vi "CountDown.vi"(10 "Cluster":T1) -> (2 "Cluster 2":T1)   [LabVIEW 2010]
uses:
  DataCluster.ctl
panel:
  out "Zero":bool
  out "Gauge":dbl(knob)
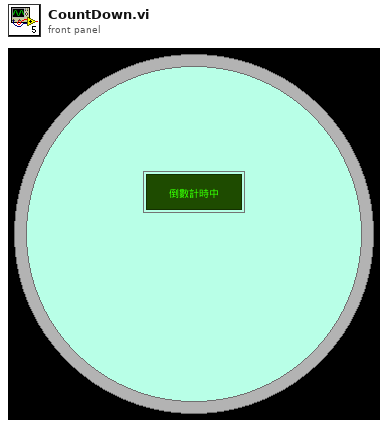
[diagram p1: front panel]
types:
  T1 = typedef "DataCluster.ctl" = cluster{"鬧鐘時間":timestamp, "鈴聲":path, "error ":errorcluster, "Min":dbl, "Sec":dbl, "鬧鐘作用":bool}
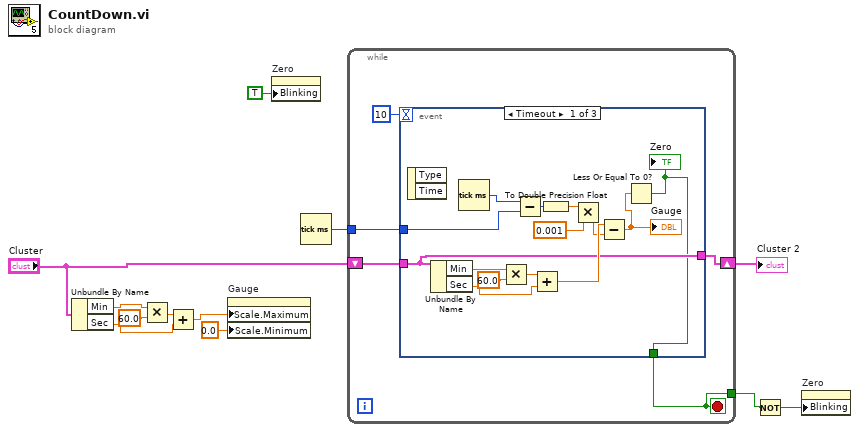
[diagram p0: block diagram]
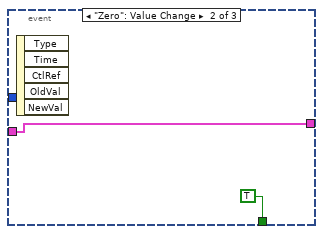
[diagram p2: hidden frame]
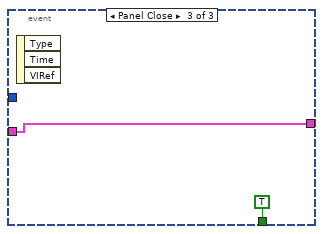
[diagram p3: hidden frame]
diagram:
  n1 = Unbundle By Name("Cluster") -> ("Min"=w4:dbl, "Sec"=w7:dbl)
  n2 = Multiply(x=w4, y=60.0) -> (x*y=w3:dbl)
  n3 = Add(x=w3, y=w7) -> (x+y=w2:dbl)
  n4 = property on="Gauge" class="Knob (strict)"("Scale.Maximum"=w2, "Scale.Minimum"=0.0 ("Scale.Range:Minimum")) -> ()  [unwired: 2 in, 2 out]
  n5 = property on="Zero" class="Bool (strict)"("Blinking"=TRUE) -> ()  [unwired: 2 in, 2 out]
  n6 = Tick Count (ms)() -> (millisecond timer value=w11:u32)
  n7 = while {
    shift-right: [w14] -> w10
    shift-left: "Cluster" -> [w16]
    tunnel: w11 -> [w15]
    tunnel: [w13] -> w8
    stop <- w13 stop-if-true
    n8 = event shown="[0] Timeout" {
      selector: _ -> [_ _ _]
      dyn-events: _ -> [_ _ _]
      timeout: 10 -> [_ _ _]
      tunnel: w16 -> [w20 w33 w35]
      tunnel: w15 -> [w26 _ _]
      tunnel: [w20 w33 w35] -> w14
      tunnel: [w18 TRUE TRUE] -> w13
      event Timeout {
        n9 = event-data() -> ()  [unwired: 1 in, 2 out]
        n10 = Unbundle By Name(w20) -> ("Min"=w31:dbl, "Sec"=w28:dbl)
        n11 = Tick Count (ms)() -> (millisecond timer value=w27:u32)
        n12 = Multiply(x=w31, y=60.0) -> (x*y=w29:dbl)
        n13 = Subtract(x=w27, y=w26) -> (x-y=w23:u32)
        n14 = Add(x=w29, y=w28) -> (x+y=w25:dbl)
        n15 = To Double Precision Float(number=w23) -> (double precision float=w22:dbl)
        n16 = Multiply(x=w22, y=0.001) -> (x*y=w21:dbl)
        n17 = Subtract(x=w25, y=w21) -> (x-y=w19:dbl)
        "Gauge" <- w19
        n18 = Less Or Equal To 0?(x=w19) -> (x <= 0?=w18:bool)
        "Zero" <- w18
      }
      event "Zero": Value Change {
        n19 = event-data() -> ()  [unwired: 1 in, 5 out]
      }
      event Panel Close {
        n20 = event-data() -> ()  [unwired: 1 in, 3 out]
      }
    }
  }
  "Cluster 2" <- w10
  n21 = Not(x=w8) -> (.not. x?=w9:bool)
  n22 = property on="Zero" class="Bool (strict)"("Blinking"=w9) -> ()  [unwired: 2 in, 2 out]
